vi "Save File Create and Check Nested Folder.vi"(8 "error in (no error)":errorcluster, 10 "Prevent Startup File":bool, 11 "Extracted File Name":path) -> (0 "error out":errorcluster, 2 "File Path":path, 3 "Base Path":path)   [LabVIEW 2023, in "Save File.lvlib"]
uses:
  Save File.lvlib
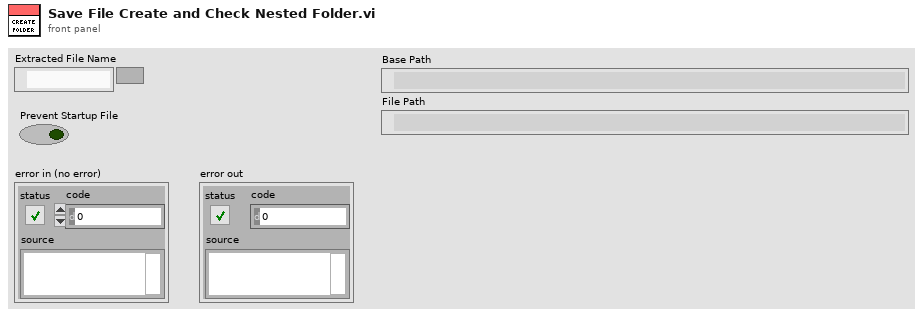
[diagram p1: front panel]
types:
  T1 = enum16{"open", "replace", "create", "open or create", "replace or create", "replace or create with confirmation"}
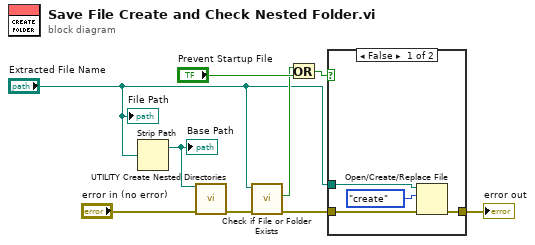
[diagram p0: block diagram]
diagram:
  n1 = Strip Path(path="Extracted File Name") -> (stripped path=w3:path)  [unwired: 1 out]
  "Base Path" <- w3
  n2 = call "UTILITY Create Nested Directories.vi"("path to create"=w3, "error in"="error in (no error)") -> ("error out"=w4:errorcluster)  [unwired: 11 in, 2 out]
  n3 = call <vilib>:"Check if File or Folder Exists.vi"("error in (no error)"=w4, "path"="Extracted File Name") -> ("error out"=w2:errorcluster, "file or folder exists?"=w7:bool)  [unwired: 7 in, 1 out]
  n4 = Or(x=w7, y="Prevent Startup File") -> (x .or. y?=w9:bool)
  n5 = case shown="False" w9 {
    tunnel: "Extracted File Name" -> [w13 _]
    tunnel: w2 -> [w11 w14]
    tunnel: [w10 w14] -> w1
    frame False {
      n6 = Open/Create/Replace File(file path (use dialog)=w13, error in=w11, operation (0:open)=T1."create") -> (error out=w10:errorcluster)  [unwired: 3 in, 2 out]
    }
    frame True {
    }
  }
  "error out" <- w1
  "File Path" <- "Extracted File Name"
